vi "Create Random Request ID.vi"(3 "Message Loop Shift Register Data (in)":T1) -> (0 "Generated Request ID":u64, 1 "Message Loop Shift Register Data (out)":T1)   [LabVIEW 2020, in "wamplv.lvlib"]
uses:
  WAMP Client.lvclass/WAMP Client.ctl
  wamplv.lvlib
  <vilib>/numeric/Random Number (Range) U64.vi
  29bcbb0d-03a8-4097-9ca0-1d3c1ec93cac.vi
  TypeDef/Publish Requests Map.ctl
  TypeDef/Endpoint Data.ctl
  TypeDef/CALL Request Map.ctl
  TypeDef/SUBSCRIBE Requests Map.ctl
  TypeDef/Subscriptions Map.ctl
  TypeDef/Unsubscribe Requests Map.ctl
  TypeDef/Message Loop Data.ctl
  TypeDef/Unregister requests map.ctl
  Private/Requests/Call/ICallRequest/ICallRequest.lvclass
  Private/Requests/Subscribe/ISubscribe/ISubscribe.lvclass
  Private/Requests/Publish/IPublish/IPublish.lvclass
  Private/Message loop classes/Subscription details/SubscriptionDetailsParent/SubscriptionDetailsParent.lvclass
  Private/Requests/Unsubscribe/IUnsubscribe/IUnsubscribe.lvclass
  Private/Requests/Register/IRegister/IRegister.lvclass
  Private/Requests/Unregister/IUnregister/IUnregister.lvclass
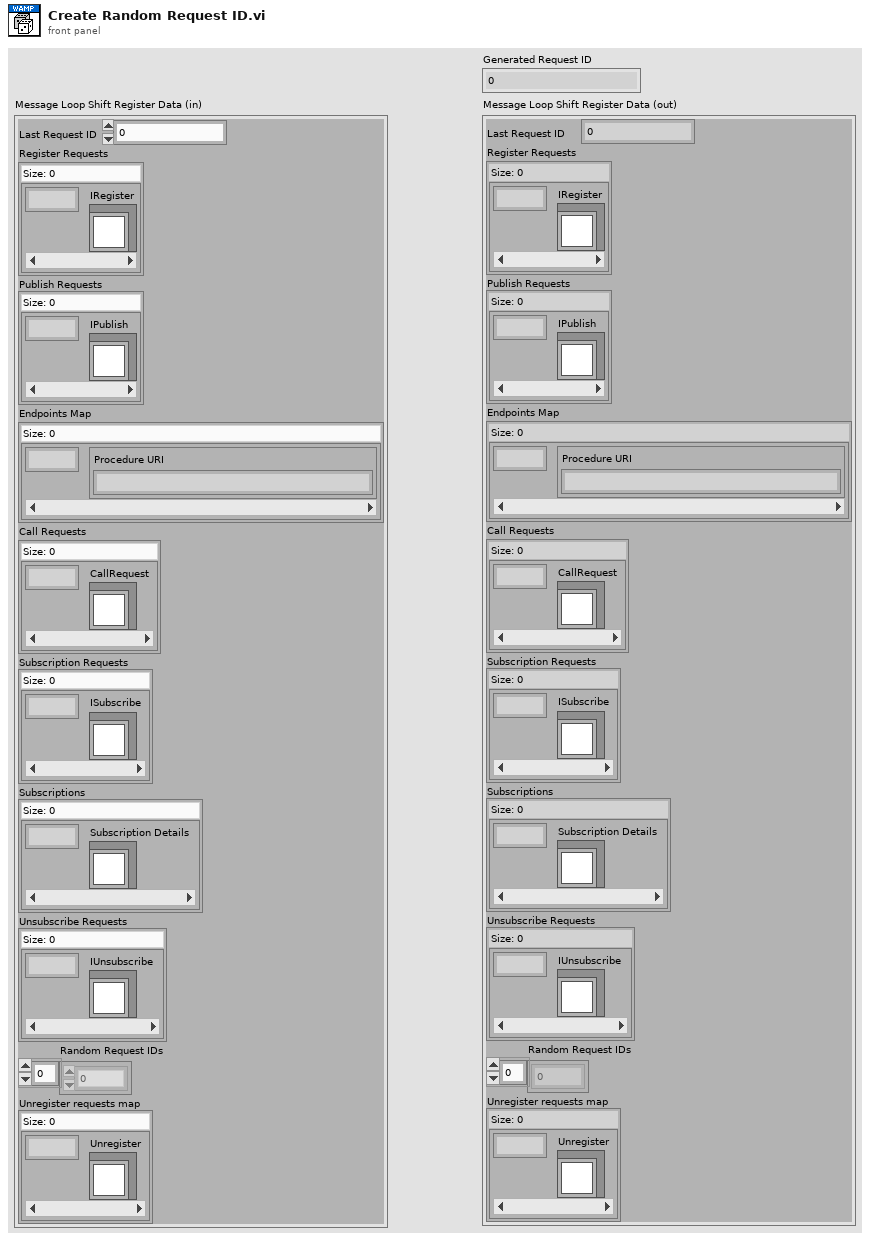
[diagram p1: front panel]
types:
  T1 = typedef "wamplv.lvlib/Message Loop Data.ctl" = cluster{"Last Request ID":u64, "Register Requests":map{u64, refnum<class "IRegister.lvclass">}, "Publish Requests":T2, "Endpoints Map":map{u64, T3}, "Call Requests":T4, "Subscription Requests":T5, "Subscriptions":T6, "Unsubscribe Requests":T7, "Random Request IDs":u64[], "Unregister requests map":T8}
  T2 = typedef "wamplv.lvlib/Publish Requests Map.ctl" = map{u64, refnum<class "IPublish.lvclass">}
  T3 = typedef "wamplv.lvlib/Endpoint Data.ctl" = cluster{"Procedure URI":string}
  T4 = typedef "wamplv.lvlib/CALL Request Map.ctl" = map{u64, refnum<class "ICallRequest.lvclass">}
  T5 = typedef "wamplv.lvlib/SUBSCRIBE Requests Map.ctl" = map{u64, refnum<class "ISubscribe.lvclass">}
  T6 = typedef "wamplv.lvlib/Subscriptions Map.ctl" = map{u64, refnum<class "SubscriptionDetailsParent.lvclass">}
  T7 = typedef "wamplv.lvlib/Unsubscribe Requests Map.ctl" = map{u64, refnum<class "IUnsubscribe.lvclass">}
  T8 = typedef "wamplv.lvlib/Unregister requests map.ctl" = map{u64, refnum<class "IUnregister.lvclass">}
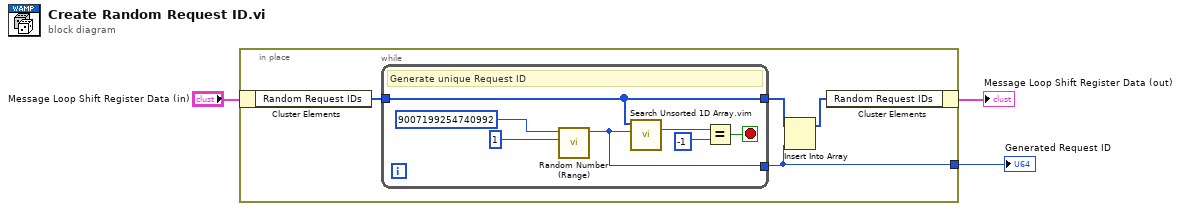
[diagram p0: block diagram]
diagram:
  n1 = in-place "In Place Element Structure" {
    in-place-border: [w4] -> w2
    n2 = in-place-cluster #1("Message Loop Shift Register Data (in)") -> ("Random Request IDs"=w6:u64[])
    n3 = while {
      tunnel: w6 -> [w8]
      tunnel: [w9] -> w4
      tunnel: [w8] -> w7
      stop <- w11 stop-if-true
      # "Generate unique Request ID"
      n4 = call-poly <vilib>:"Random Number (Range).vi"("lower bound (0)"=u64 1, "upper bound (100)"=u64 9007199254740992) -> ("number"=w9:u64)  [unwired: 9 in]
      n5 = call "Search Unsorted 1D Array.vim"("element"=w9, "unsorted 1D array"=w8) -> ("index of element"=w10:i32)  [unwired: 9 in]
      n6 = Equal?(x=w10, y=-1) -> (x = y?=w11:bool)
    }
    n7 = Insert Into Array(array=w7, new element=w4) -> (w5:u64[])  [unwired: 1 in]
    n8 = in-place-cluster #1("Random Request IDs"=w5) -> (→"Message Loop Shift Register Data (out)":T1)
  }
  "Generated Request ID" <- w2
